vi "Init Data.vi"(8 "error in (no error)":errorcluster, 11 "Rigol DG822 Pulse in":refnum<class "Rigol DG822 Pulse.lvclass">) -> (0 "error out":errorcluster, 3 "Rigol DG822 Pulse out":refnum<class "Rigol DG822 Pulse.lvclass">)   [LabVIEW 2021, in "Rigol DG822 UI.lvlib" / "Rigol DG822 Pulse.lvlib" / "Rigol DG822 Pulse.lvclass"]
uses:
  Rigol DG822 Pulse.lvclass
  Rigol DG822 Pulse.lvclass/Rigol DG822 Pulse.ctl
  General/Files/lvlibp/Actors.lvlibp/Actors/Actors/Actors.lvclass
  D:/LabVIEW/General/Files/lvlibp/Actors.lvlibp/Actors/Actors/Actors.lvclass
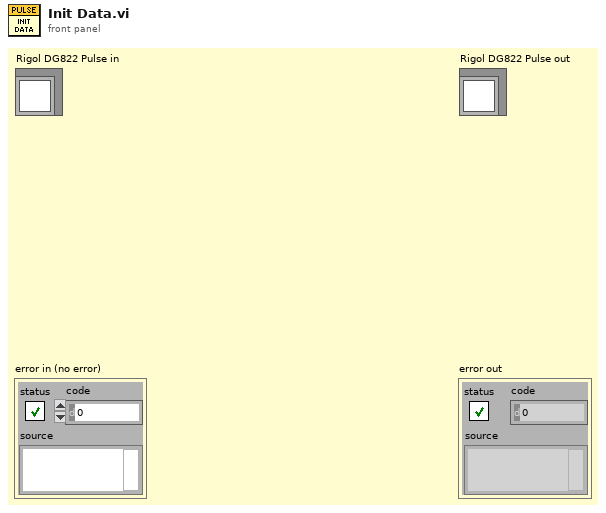
[diagram p1: front panel]
types:
  T1 = cluster{"Freq-Period":string, "Freq-Period 2":string, "Freq-Period 3":string, "Freq-Period 4":string, "Freq-Period 5":string, "Freq-Period 6":string, "Freq-Period 7":string}
  T2 = cluster{"Control Label 5":string, "Control Label 6":string, "Control Label":string, "Control Label 2":string, "Control Label 3":string, "Control Label 4":string, "Control Label 7":string, "Control Label 8":string, "Control Label 9":string}
  T3 = cluster{"Control Label":string, "Control Label 2":string, "Control Label 3":string, "Control Label 4":string}
  T4 = typedef "FT Controls Cluster.ctl" = cluster{"Freq/Period":bool, "Ampl/HighL":bool, "Offset/LowL":bool, "Duty/Width":bool}
  T5 = typedef "String Indicators Cluster.ctl" = cluster{"Freq-Period":string, "Ampl-HighL":string, "Offset-LowL":string, "Phase":string, "Duty-Width":string, "RisEdge":string, "FallEdge":string}
  T6 = enum32{"No Selection", "MHz", "kHz", "Hz", "mHz", "uHz"}
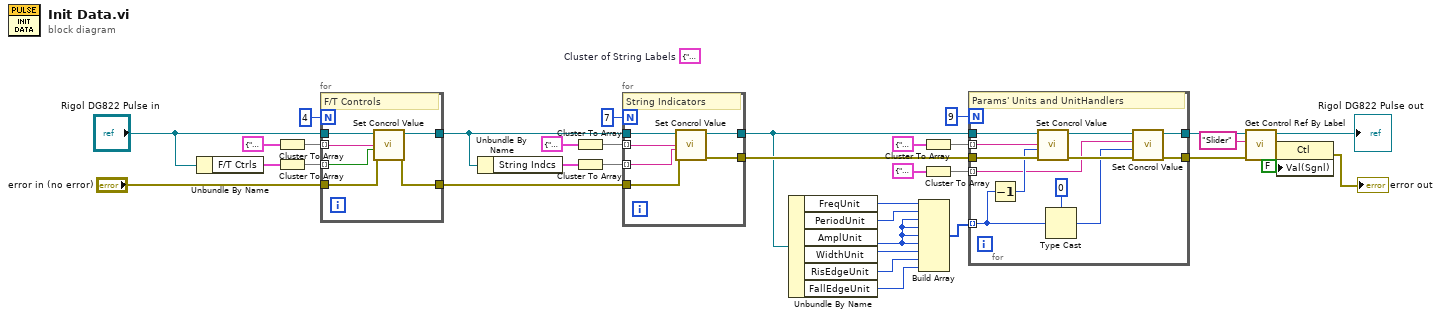
[diagram p0: block diagram]
diagram:
  (unwired) T1 {"Freq-Period"="String Indcs.Freq-Period", "Freq-Period 2"="String Indcs.Ampl-HighL", "Freq-Period 3"="String Indcs.Offset-LowL", "Freq-Period 4"="String Indcs.Phase", "Freq-Period 5"="String Indcs 2.Duty-Width", "Freq-Period 6"="String Indcs 2.RisEdge", "Freq-Period 7"="String Indcs 2.Falldge"}  # Cluster of String Labels
  n1 = Unbundle By Name("Rigol DG822 Pulse in") -> ("F/T Ctrls"=w31:T4)
  n2 = Cluster To Array(cluster=T3 {"Control Label"="F/T Ctrls.Freq/Period", "Control Label 2"="F/T Ctrls.Ampl/HighL", "Control Label 3"="F/T Ctrls.Offset/LowL", "Control Label 4"="F/T Ctrls 2.Duty/Width"}) -> (array=w29:string[])
  n3 = Cluster To Array(cluster=w31) -> (array=w28:bool[])
  n4 = for {
    N: 4 -> [_]
    tunnel: w29 -> [w42] mode=indexing
    tunnel: "Rigol DG822 Pulse in" -> [w41]
    tunnel: w28 -> [w40] mode=indexing
    tunnel: "error in (no error)" -> [w39]
    tunnel: [w38] -> w25
    tunnel: [w37] -> w21
    # "F/T Controls"
    n5 = call "Set Concrol Value.vi"("error in (no error)"=w39, "Value"=w40, "Control Label"=w42, "Actors in"=w41) -> ("error out"=w38:errorcluster, "Actors out"=w37:refnum<class "Rigol DG822 Pulse.lvclass">)  [unwired: 6 in]
  }
  n6 = Unbundle By Name(w21) -> ("String Indcs"=w24:T5)
  n7 = Cluster To Array(cluster=T1 {"Freq-Period"="String Indcs.Freq-Period", "Freq-Period 2"="String Indcs.Ampl-HighL", "Freq-Period 3"="String Indcs.Offset-LowL", "Freq-Period 4"="String Indcs.Phase", "Freq-Period 5"="String Indcs 2.Duty-Width", "Freq-Period 6"="String Indcs 2.RisEdge", "Freq-Period 7"="String Indcs 2.FallEdge"} ("Cluster of String Labels")) -> (array=w22:string[])
  n8 = Cluster To Array(cluster=w24) -> (array=w23:string[])
  n9 = for {
    N: 7 -> [_]
    tunnel: w22 -> [w48] mode=indexing
    tunnel: w21 -> [w47]
    tunnel: w23 -> [w46] mode=indexing
    tunnel: w25 -> [w45]
    tunnel: [w44] -> w19
    tunnel: [w43] -> w17
    # "String Indicators"
    n10 = call "Set Concrol Value.vi"("error in (no error)"=w45, "Value"=w46, "Control Label"=w48, "Actors in"=w47) -> ("error out"=w44:errorcluster, "Actors out"=w43:refnum<class "Rigol DG822 Pulse.lvclass">)  [unwired: 6 in]
  }
  n11 = Unbundle By Name(w17) -> ("FreqUnit"=w16:T6, "PeriodUnit"=w14:enum32{"No Selection", "s", "ms", "us", "ns"}, "AmplUnit"=w15:enum32{"No Selection", "Vpp", "mVpp"}, "WidthUnit"=w11:enum32{"No Selection", "s", "ms", "us", "ns"}, "RisEdgeUnit"=w10:enum32{"No Selection", "s", "ms", "us", "ns"}, "FallEdgeUnit"=w9:enum32{"No Selection", "s", "ms", "us", "ns"})
  n12 = Build Array(w16, w14, w15, w15, w15, w15, w11, w10, w9) -> (w18:u32[])
  n13 = Cluster To Array(cluster=T2 {"Control Label 5"="FreqUnitHandler", "Control Label 6"="PeriodUnitHandler", "Control Label"="AmplUnitHandler", "Control Label 2"="HighLUnitHandler", "Control Label 3"="OffsetUnitHandler", "Control Label 4"="LowLUnitHandler", "Control Label 7"="WidthUnitHandler", "Control Label 8"="RisEdgeUnitHandler", "Control Label 9"="FallEdgeUnitHandler"}) -> (array=w34:string[])
  n14 = Cluster To Array(cluster=T2 {"Control Label 5"="FreqUnit", "Control Label 6"="PeriodUnit", "Control Label"="AmplUnit", "Control Label 2"="HighLUnit", "Control Label 3"="OffsetUnit", "Control Label 4"="LowLUnit", "Control Label 7"="WidthUnit", "Control Label 8"="RisEdgeUnit", "Control Label 9"="FallEdgeUnit"}) -> (array=w32:string[])
  n15 = for {
    N: 9 -> [_]
    tunnel: w17 -> [w59]
    tunnel: [w57] -> w3
    tunnel: [w56] -> w2
    tunnel: w19 -> [w55]
    tunnel: w34 -> [w54] mode=indexing
    tunnel: w32 -> [w52] mode=indexing
    tunnel: w18 -> [w49] mode=indexing
    # "Params' Units and UnitHandlers"
    n16 = Decrement(x=w49) -> (x-1=w53:u32)
    n17 = call "Set Concrol Value.vi"("error in (no error)"=w55, "Value"=w53, "Control Label"=w54, "Actors in"=w59) -> ("error out"=w60:errorcluster, "Actors out"=w58:refnum<class "Rigol DG822 Pulse.lvclass">)  [unwired: 6 in]
    n18 = Type Cast(type=0, x=w49) -> (*(type *) &x=w51:i32)
    n19 = call "Set Concrol Value.vi"("error in (no error)"=w60, "Value"=w51, "Control Label"=w52, "Actors in"=w58) -> ("error out"=w56:errorcluster, "Actors out"=w57:refnum<class "Rigol DG822 Pulse.lvclass">)  [unwired: 6 in]
  }
  n20 = call "Get Control Ref By Label.vi"("error in (no error)"=w2, "Control Label"="Slider", "Actors in"=w3) -> ("error out"=w6:errorcluster, "Control Ref"=w7:refnum<vi>, "Actors out"=→"Rigol DG822 Pulse out":refnum<class "Rigol DG822 Pulse.lvclass">)  [unwired: 6 in]
  n21 = property class="Ctl"(reference=w7, error in=w6, "Val(Sgnl)"=FALSE) -> (error out=→"error out":errorcluster)  [unwired: 1 out]
